vi "Read Address.vi"(7 "Actor":refnum<class "Actor.lvclass">) -> (2 "Address":refnum<data-value>)   [LabVIEW 2020, in "jettl.lvlib" / "Queue Transport.lvlib"]
uses:
  Queue Transport.lvlib
  Queue Transport/Queue Transport.lvclass
  Read Self Attributes/Read Self Attributes.lvlib
  Read Self Attributes/Transport.vi
  Actor/Actor.lvclass
  Relation.ctl
  jettl.lvlib
  Teller.ctl
  Msg Attributes.ctl
  Msg Input/Msg Input.lvclass
  Msg Output/Msg Output.lvclass
  Msg/Msg.lvclass
  Transport/Transport.lvclass
  Msgs.ctl
  Unified Layer.ctl
  Actor Attributes.ctl
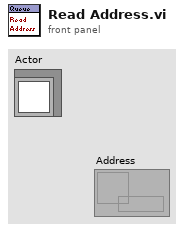
[diagram p1: front panel]
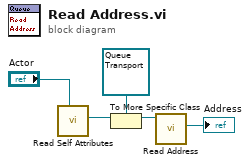
[diagram p0: block diagram]
diagram:
  n1 = call-poly "Read Self Attributes.vi"("Actor in"="Actor") -> ("Transport"=w3:refnum<class "Transport.lvclass">)  [unwired: 10 in]
  n2 = To More Specific Class(target class=refnum<class "Queue Transport.lvclass"> refnum ("jettl.lvlib:Transport.lvlib:Queue Transport.lvclass"), reference=w3) -> (specific class reference=w4:refnum<class "Queue Transport.lvclass">)  [unwired: 1 in, 1 out]
  n3 = call "Read Address.vi"("Queue Transport in"=w4) -> ("Address"=→"Address":refnum<data-value>)  [unwired: 10 in]
